vi "Clear Snap GUI.vi"(8 "error in (no error)":errorcluster, 11 "4300 in":refnum<class "4300.lvclass">) -> (0 "error out":errorcluster, 3 "4300 out":refnum<class "4300.lvclass">)   [LabVIEW 2019, in "4300.lvlib" / "4300.lvclass"]
uses:
  Library/4300.lvclass
  C:/Users/Public/Documents/Development/builds/Instruments/Instruments.lvlibp/Library/Instruments.lvclass
  builds/Instruments/Instruments.lvlibp/Accessors/Read Snapshot Refnum.vi
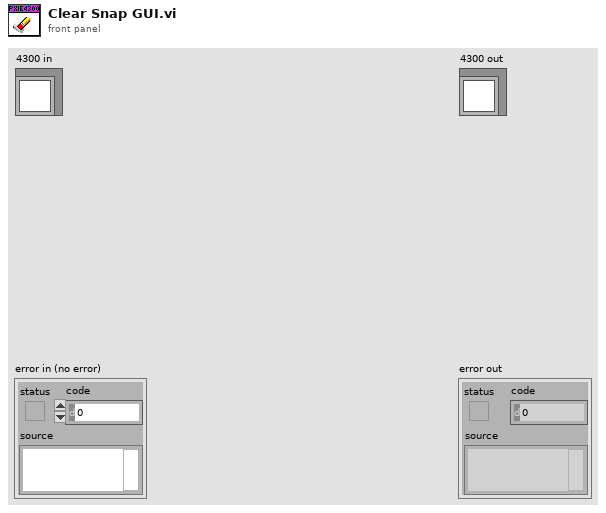
[diagram p1: front panel]
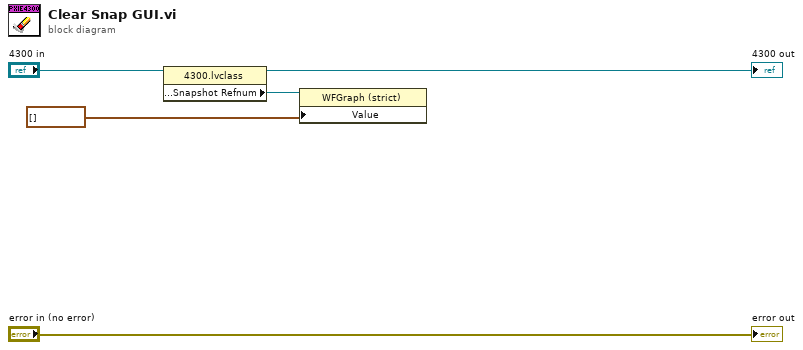
[diagram p0: block diagram]
diagram:
  n1 = property class="4300.lvclass"(reference="4300 in") -> (reference out=→"4300 out":refnum<class "4300.lvclass">, "Accessors:GUI:Snapshot Refnum"=w3:refnum<vi>)  [unwired: 1 in, 1 out]
  n2 = property class="WFGraph (strict)"(reference=w3, "Value"=waveform(dbl)[] []) -> ()  [unwired: 1 in, 2 out]
  "error out" <- "error in (no error)"
